vi "Read Discrete Input Channels.vi"(8 "error in (no error)":errorcluster, 9 "Discrete Inputs in":T1[](array[typedef]), 11 "Modbus Master in":refnum<class "Modbus Master.lvclass">) -> (0 "error out":errorcluster, 2 "Discrete Input Data Out":dbl[](array[numeric]), 3 "Modbus Master out":refnum<class "Modbus Master.lvclass">)   [LabVIEW 2015]
uses:
  Modbus API.lvlibp/API/Master/Modbus Master.lvclass
  Shared/Controls/Data Model/Channel.ctl
  System Explorer/SubVIs/Modbus Type.ctl
  <vilib>/NI Veristand/Custom Device API/Custom Device Channel Type.ctl
  Shared/Controls/Data Model/Mapping.ctl
  Shared/Controls/Data Model/DataType.ctl
  <vilib>/NI Veristand/Custom Device API/Custom Device Item Ref.ctl
  Shared/Modbus Master Shared.lvlib
  <vilib>/NI VeriStand/Custom Device API/Custom Device API.lvlib
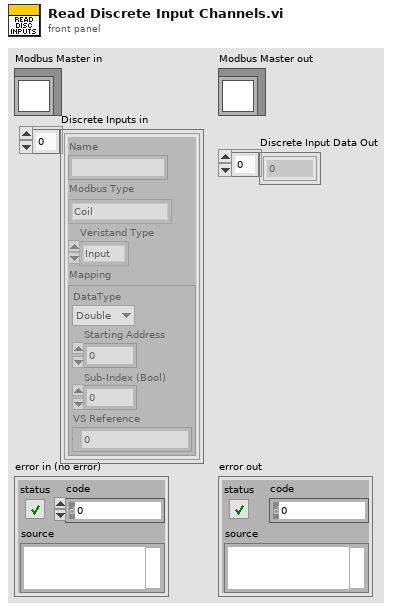
[diagram p1: front panel]
types:
  T1 = typedef "Modbus Master Shared.lvlib/Channel.ctl" = cluster{"Name":string, "Modbus Type":T2, "Veristand Type":T3, "Mapping":T4}
  T2 = typedef "Modbus Master Shared.lvlib/Modbus Type.ctl" = enum16{"Coil", "Discrete Input", "Holding Register", "Input Register"}
  T3 = typedef "Custom Device API.lvlib/Custom Device Channel Type.ctl" = enum16{"Input", "Output"}
  T4 = typedef "Modbus Master Shared.lvlib/Mapping.ctl" = cluster{"DataType":T5, "Starting Address":u16, "Sub-Index (Bool)":u16, "VS Reference":T6}
  T5 = typedef "Modbus Master Shared.lvlib/DataType.ctl" = enum16{"Double", "Single", "I64", "I32", "I16", "I8", "U64", "U32", "U16", "U8", "Boolean"}
  T6 = typedef "Custom Device API.lvlib/Custom Device Item Ref.ctl" = u64
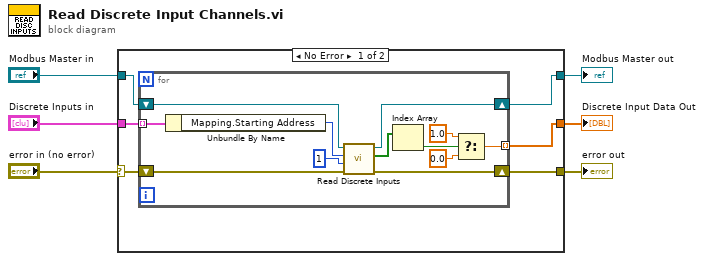
[diagram p0: block diagram]
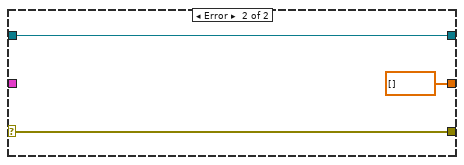
[diagram p2: hidden frame]
diagram:
  n1 = case shown="No Error" "error in (no error)" {
    selector: "error in (no error)" -> [w10 w27]
    tunnel: [w12 w25] -> w6
    tunnel: "Modbus Master in" -> [w11 w25]
    tunnel: "Discrete Inputs in" -> [w9 _]
    tunnel: [w8 w27] -> w2
    tunnel: [w7 dbl[] []] -> w1
    frame No Error {
      n2 = for {
        shift-right: [w20] -> w8
        shift-left: w10 -> [w21]
        tunnel: w9 -> [w24] mode=indexing
        shift-right: [w22] -> w12
        shift-left: w11 -> [w23]
        tunnel: [w13] -> w7 mode=indexing
        n3 = Unbundle By Name(w24) -> ("Mapping.Starting Address"=w19:u16)
        n4 = call-dynamic "Read Discrete Inputs.vi"("error in"=w21, "number of inputs"=u16 1, "starting address"=w19, "Modbus master in"=w23) -> ("error out"=w20:errorcluster, "discrete inputs"=w17:bool[], "Modbus master out"=w22:refnum<class "Modbus Master.lvclass">)  [unwired: 5 in]
        n5 = Index Array(array=w17) -> (element=w16:bool)  [unwired: 1 in]
        n6 = Select(t=1.0, s=w16, f=0.0) -> (s? t:f=w13:dbl)
      }
    }
    frame Error {
    }
  }
  "Discrete Input Data Out" <- w1
  "Modbus Master out" <- w6
  "error out" <- w2
